vi "RT_PWM_dc_motor.vi"() -> ()   [LabVIEW 2019]
uses:
  <vilib>/FPGAPlugInAG/myRIO-1900/niLvFpga_Open_myRIO-1900.vi
  <vilib>/rvi/interface/common/dynamic/niFpgaDynamicAddResources.vi
  <vilib>/Utility/error.llb/Error Cluster From Error Code.vi
  <vilib>/rvi/errors/niLvFpgaAdjustHostInterfaceError.vi
  <vilib>/addons/control/pid/pid.llb/PID Advanced (DBL).vi
  <vilib>/FPGAPlugInAG/Dynamic/niLvFpga_Close_Dynamic.vi
  <vilib>/rvi/interface/nirviOpenFPGA/nirviOpenFPGA.xnode
  FPGA Bitfiles/gpass2_FPGATarget_FPGAPWMdcmotor_MgAzi-ogCtI.lvbitx
  FPGA_PWM_dc_motor.vi
  <vilib>/rvi/interface/nirviReadWriteControl/nirviReadWriteControl.xnode
  <vilib>/rvi/interface/nirviCloseFPGA/nirviCloseFPGA.xnode
  NiFpgaLv.dll
  <vilib>/rvi/interface/Simulation/niFpgaSimulationCallBeginRW.vi
  <vilib>/addons/control/pid/NI_PID_pid.lvlib
panel:
  out "measured velocity [rev/s]":dbl
  out "rev/tick":dbl
  in  "Control mode":enum16{"Stop", "Closed Loop", "Manual"}(ring)
  in  "DC PWM Frequency (Hz)":sgl
  out "pwm output":i16
  in  "reinitialize? (F)":bool
  in  "PID gains":T1={"proportional gain (Kc)"=1.0101010101010102, "integral time (Ti, min)"=0.00808080808080808, "derivative time (Td, min)"=0.0} {"derivative time (Td, min)" scale=0.0..10.0; "integral time (Ti, min)" scale=0.0..0.2; "proportional gain (Kc)" scale=0.0..10.0}
  out "controller pwm output":i16(graph)
  in  "setpoint":i16(slide) scale=-200.0..200.0
  out "velocity":dbl(graph)
  in  "stop":bool
  in  "Controller PWM output [-100,100]%":i16(slide) scale=-100.0..100.0
  out "Position (Counts)":i64
  out "Acceleration (Counts/Interval)":i32
  out "Velocity (Counts/Interval)":i32
  in  "Loop Timer DAQ":u32=1
  in  "Position Reset":bool
  in  "Velocity Interval (uSec)":u32=1000
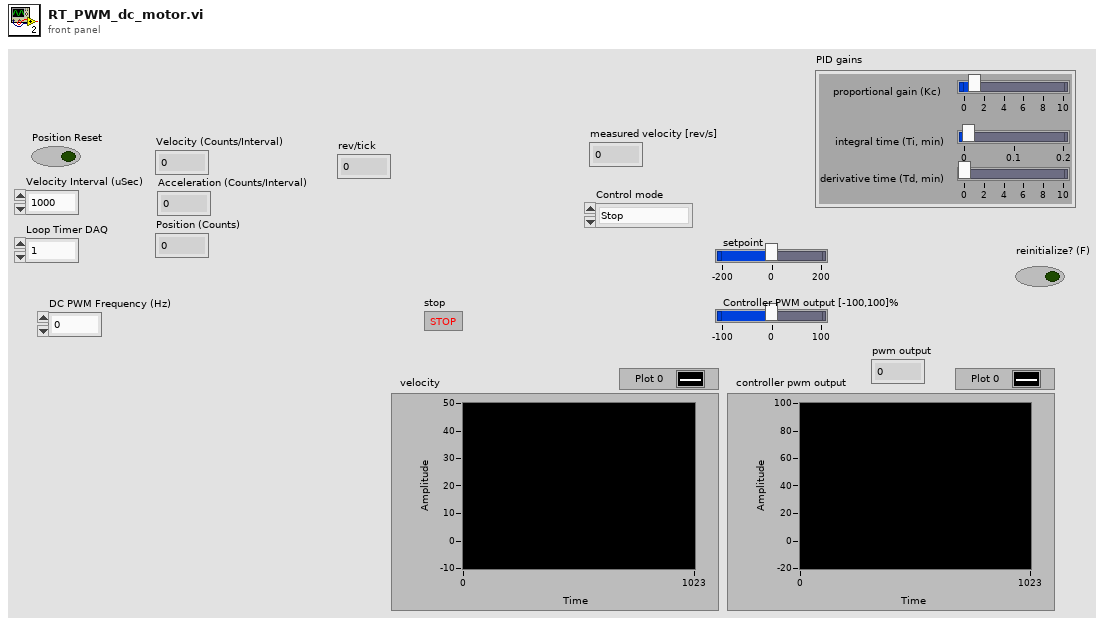
[diagram p1: front panel]
types:
  T1 = cluster{"proportional gain (Kc)":dbl, "integral time (Ti, min)":dbl, "derivative time (Td, min)":dbl}
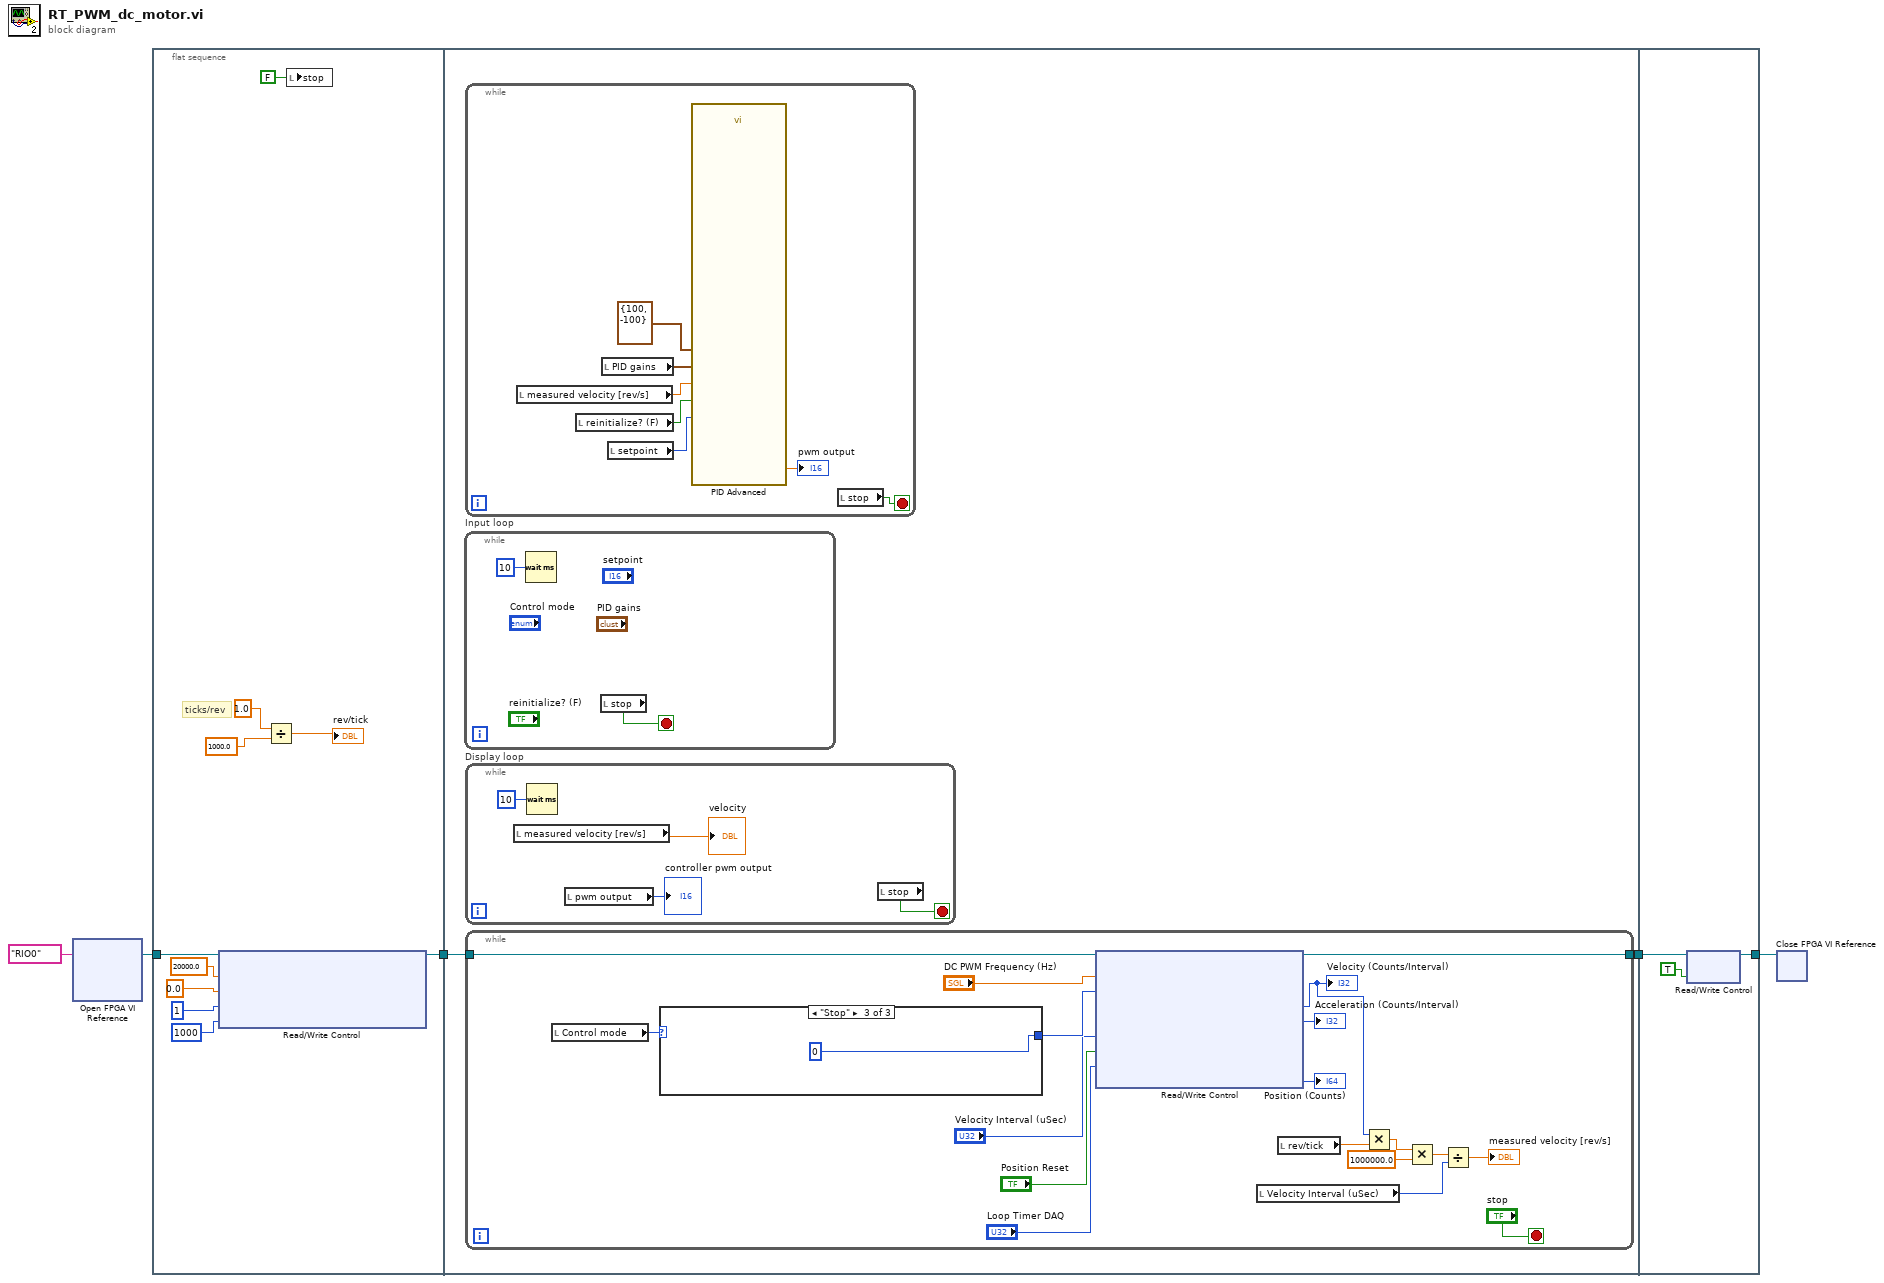
[diagram p0: block diagram]
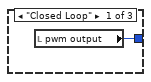
[diagram p2: hidden frame]
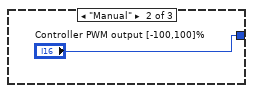
[diagram p3: hidden frame]
diagram:
  n1 = xnode "Open FPGA VI Reference"("resource name"=tag "RIO0") -> ("FPGA VI Reference Out"=w4:refnum<k20>)  [unwired: 1 in, 1 out]
  n2 = flat-sequence {
    tunnel: w4 -> [w15]
    tunnel: [w12] -> w3
    tunnel: w3 -> [w17]
    tunnel: [w16] -> w1
    tunnel: [w53] -> w2
    tunnel: w1 -> [w52]
    frame #0 {
      # "ticks/rev"
      n3 = xnode "Read/Write Control"("FPGA VI Reference In"=w15, "DC PWM Frequency (Hz)"=sgl 20000.0, "Controller PWM output [-100,100]%"=sgl 0.0, "Loop Timer DAQ"=u32 1, "Velocity Interval (uSec)"=u32 1000) -> ("FPGA VI Reference Out"=w12:refnum<k20>)  [unwired: 1 in, 1 out]
      n4 = Divide(x=1.0, y=1000.0) -> (x/y=→"rev/tick":dbl)
      n5 = local write "stop"(FALSE ("stop")) -> ()
    }
    frame #1 {
      n6 = while "Input loop" {
        stop <- w25 stop-if-true
        n7 = Wait (ms)(milliseconds to wait=u32 10) -> ()  [unwired: 1 out]
        n8 = local read "stop"() -> (w25:bool)
      }
      n9 = while {
        stop <- w18 stop-if-true
        n10 = local read "measured velocity [rev/s]"() -> (w20:dbl)
        n11 = local read "reinitialize? (F)"() -> (w21:bool)
        n12 = local read "PID gains"() -> (w24:T1)
        n13 = local read "setpoint"() -> (w22:i16)
        n14 = call-poly <vilib>:"PID Advanced.vi"("setpoint"=w22, "output range"=cluster{"output high":i8, "output low":i8} {"output high"=100, "output low"=-100}, "process variable"=w20, "PID gains"=w24, "reinitialize? (F)"=w21) -> ("output"=→"pwm output":dbl)  [unwired: 9 in, 1 out]
        n15 = local read "stop"() -> (w18:bool)
      }
      n16 = while "Display loop" {
        stop <- w29 stop-if-true
        n17 = local read "measured velocity [rev/s]"() -> (→"velocity":dbl)
        n18 = Wait (ms)(milliseconds to wait=u32 10) -> ()  [unwired: 1 out]
        n19 = local read "pwm output"() -> (→"controller pwm output":i16)
        n20 = local read "stop"() -> (w29:bool)
      }
      n21 = while {
        tunnel: w17 -> [w48]
        tunnel: [w38] -> w16
        stop <- "stop" stop-if-true
        n22 = local read "Control mode"() -> (w46:enum16{"Stop", "Closed Loop", "Manual"})
        n23 = case shown="\"Stop\"" w46 {
          tunnel: [w49 "Controller PWM output [-100,100]%" i16 0] -> w45
          frame "Closed Loop" {
            n24 = local read "pwm output"() -> (w49:i16)
          }
          frame "Manual" {
          }
          frame "Stop" {
          }
        }
        n25 = xnode "Read/Write Control"("FPGA VI Reference In"=w48, "DC PWM Frequency (Hz)"="DC PWM Frequency (Hz)", "Controller PWM output [-100,100]%"=w45, "Velocity Interval (uSec)"="Velocity Interval (uSec)", "Position Reset"="Position Reset", "Loop Timer DAQ"="Loop Timer DAQ") -> ("FPGA VI Reference Out"=w38:refnum<k20>, "Velocity (Counts/Interval)"=w37:i32, "Acceleration (Counts/Interval)"=→"Acceleration (Counts/Interval)":i32, "Position (Counts)"=→"Position (Counts)":i64)  [unwired: 1 in, 1 out]
        "Velocity (Counts/Interval)" <- w37
        n26 = local read "Velocity Interval (uSec)"() -> (w32:u32)
        n27 = local read "rev/tick"() -> (w36:dbl)
        n28 = Multiply(x=w37, y=w36) -> (x*y=w35:dbl)
        n29 = Multiply(x=w35, y=1000000.0) -> (x*y=w33:dbl)
        n30 = Divide(x=w33, y=w32) -> (x/y=→"measured velocity [rev/s]":dbl)
      }
    }
    frame #2 {
      n31 = xnode "Read/Write Control"("FPGA VI Reference In"=w52, "stop"=TRUE) -> ("FPGA VI Reference Out"=w53:refnum<k20>)  [unwired: 1 in, 1 out]
    }
  }
  n32 = xnode "Close FPGA VI Reference"("FPGA VI Reference In"=w2) -> ()  [unwired: 1 in, 1 out]
